vi "Set Power Range.vi"(6 "Auto Range":bool, 8 "error in (no error)":errorcluster, 10 "Power Level":u32, 11 "2936r in":refnum<class "2936r.lvclass">) -> (0 "error out":errorcluster, 3 "2936r out":refnum<class "2936r.lvclass">)   [LabVIEW 2018, in "2936r.lvlib" / "2936r.lvclass"]
uses:
  2936r.lvclass
  2936r.lvclass/2936r.ctl
  C:/Projects/LabVIEW/Built/Optical Power Meter/2936R/Required library/PowerMeterCommands.dll
  Required library/PowerMeterCommands.dll
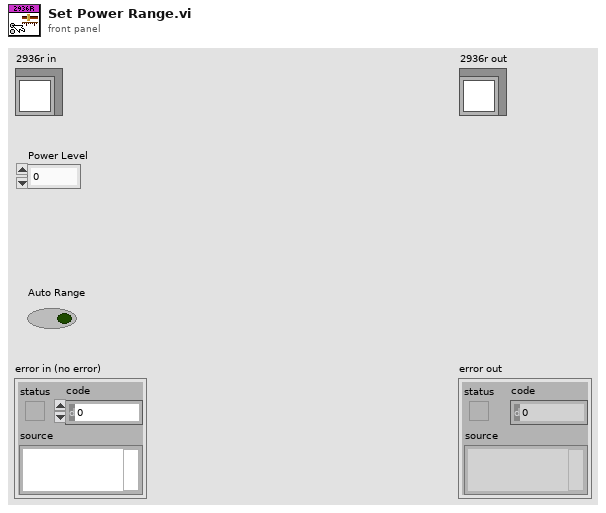
[diagram p1: front panel]
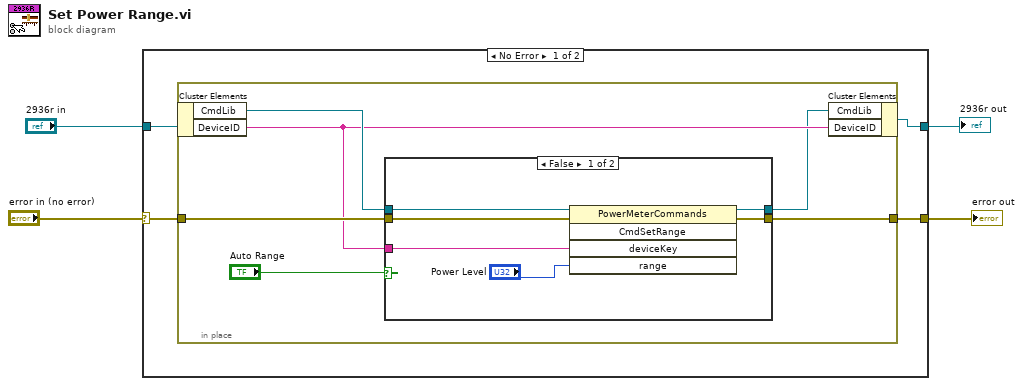
[diagram p0: block diagram]
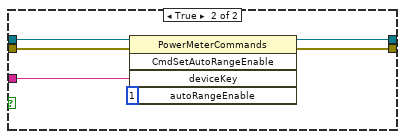
[diagram p2: hidden frame]
diagram:
  n1 = case shown="No Error" "error in (no error)" {
    selector: "error in (no error)" -> [w7 w28]
    tunnel: [w6 w28] -> w3
    tunnel: "2936r in" -> [w8 w27]
    tunnel: [w5 w27] -> w1
    frame No Error {
      n2 = in-place {
        in-place-border: w7 -> [w14]
        in-place-border: [w10] -> w6
        n3 = in-place-cluster #1(w8) -> ("CmdLib"=w13:refnum<k24>, "DeviceID"=w12:string)
        n4 = case shown="False" "Auto Range" {
          tunnel: w14 -> [w17 w26]
          tunnel: w13 -> [w20 w25]
          tunnel: w12 -> [w19 w24]
          tunnel: [w18 w23] -> w11
          tunnel: [w16 w22] -> w10
          frame False {
            n5 = invoke class="PowerMeterCommands" method="CmdSetRange"(reference=w20, error in=w17, "deviceKey"=w19, "range"="Power Level") -> (reference out=w18:refnum<k24>, error out=w16:errorcluster)  [unwired: 1 in, 3 out]
          }
          frame True {
            n6 = invoke class="PowerMeterCommands" method="CmdSetAutoRangeEnable"(reference=w25, error in=w26, "deviceKey"=w24, "autoRangeEnable"=1) -> (reference out=w23:refnum<k24>, error out=w22:errorcluster)  [unwired: 1 in, 3 out]
          }
        }
        n7 = in-place-cluster #1("CmdLib"=w11, "DeviceID"=w12) -> (w5:refnum<class "2936r.lvclass">)
      }
    }
    frame Error {
    }
  }
  "error out" <- w3
  "2936r out" <- w1
